vi "Spartan HTTP Server Error Reply.vi"(2 "message":string) -> (0 "content":string, 1 "header":string)   [LabVIEW 2011]
uses:
  <vilib>/addons/internet/http/http0.llb/HTTP LVHTTP Global.vi
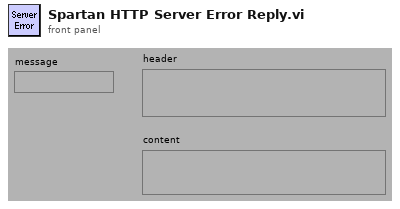
[diagram p1: front panel]
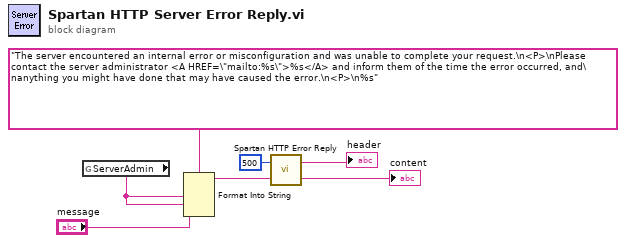
[diagram p0: block diagram]
diagram:
  n1 = global read "HTTP LVHTTP Global.vi" "ServerAdmin"() -> (w1:string)
  n2 = Format Into String(format string="The server encountered an internal error or misconfiguration and was unable to complete your request.\n<P>\nPlease contact the server administrator <A HREF=\"mailto:%s\">%s</A> and inform them of the time the error occurred, and\nanything you might have done that may have caused the error.\n<P>\n%s", w1, w1, "message") -> (resulting string=w2:string)  [unwired: 2 in, 1 out]
  n3 = call "Spartan HTTP Error Reply.vi"("message"=w2, "status code"=500) -> ("content"=→"content":string, "header"=→"header":string)
